vi "Get Test Information.vi"(8 "error in (no error)":errorcluster, 11 "Sequencer Module runtime in":refnum<class "Sequencer Module runtime.lvclass">) -> (0 "error out":errorcluster, 2 "Test Information":T1={"UUT Result"="Result", "Sequence Name"="", "Sequence Version"=""}, 3 "Sequencer Module runtime out":refnum<class "Sequencer Module runtime.lvclass">)   [LabVIEW 2015, in "Sequencer Module runtime.lvclass"]
uses:
  Sequencer Module runtime.lvclass
  classes/Report Information/Test Information.ctl
  Sequencer Module runtime.lvclass/Sequencer Module runtime.ctl
  classes/Sequence/Execution/Sequence.lvclass
  classes/Report Information/Report Information.lvclass
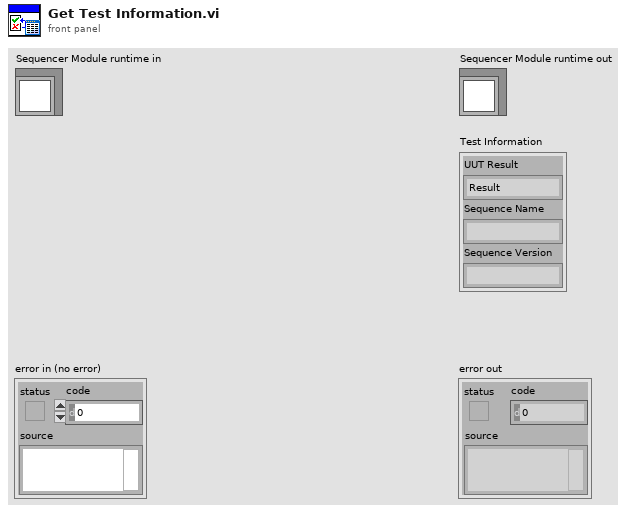
[diagram p1: front panel]
types:
  T1 = typedef "Report Information.lvclass/Test Information.ctl" = cluster{"UUT Result":string, "Sequence Name":string, "Sequence Version":string}
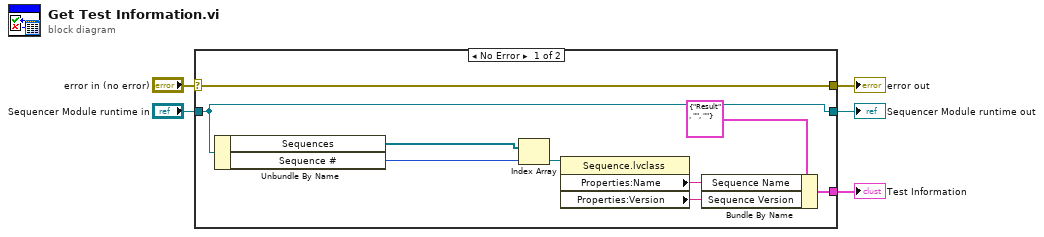
[diagram p0: block diagram]
diagram:
  n1 = case shown="No Error" "error in (no error)" {
    selector: "error in (no error)" -> [w14 w16]
    tunnel: [w14 w16] -> w4
    tunnel: [w13 w15] -> w2
    tunnel: "Sequencer Module runtime in" -> [w13 w15]
    tunnel: [w6 _] -> w1
    frame No Error {
      n2 = Unbundle By Name(w13) -> ("Sequences"=w8:refnum<class "Sequence.lvclass">[], "Sequence #"=w7:i32)
      n3 = Index Array(array=w8, index=w7) -> (element=w11:refnum<class "Sequence.lvclass">)
      n4 = property class="Sequence.lvclass"(reference=w11) -> ("Properties:Name"=w10:string, "Properties:Version"=w9:string)  [unwired: 1 in, 2 out]
      n5 = Bundle By Name(cluster=T1 {"UUT Result"="Result", "Sequence Name"="", "Sequence Version"=""} ("Test Information 2"), "Sequence Name"=w10, "Sequence Version"=w9) -> (w6:T1)
    }
    frame Error {
    }
  }
  "error out" <- w4
  "Sequencer Module runtime out" <- w2
  "Test Information" <- w1
